vi "Write Node.vi"(8 "error in (no error)":errorcluster, 10 "BT.lvlib:abs_Node.lvclass":refnum<class "abs_Node.lvclass">, 11 "abs_Decorator in":refnum<class "abs_Decorator.lvclass">) -> (0 "error out":errorcluster, 3 "abs_Decorator out":refnum<class "abs_Decorator.lvclass">)   [LabVIEW 2021, in "BT.lvlib" / "abs_Decorator.lvclass"]
uses:
  abs_Decorator.lvclass
  abs_Node/abs_Node.lvclass
  abs_Decorator.lvclass/abs_Decorator.ctl
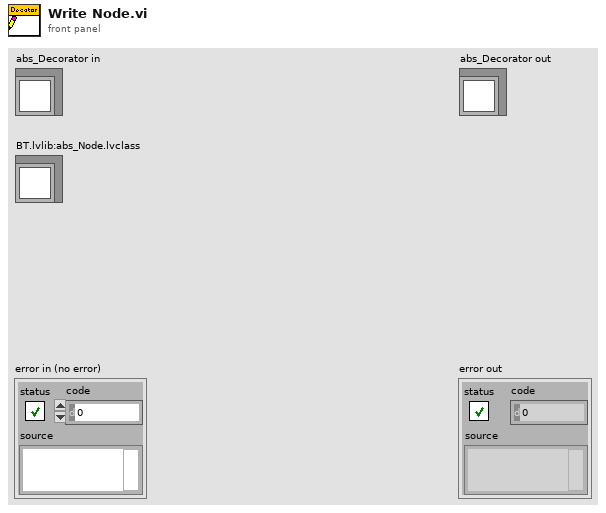
[diagram p1: front panel]
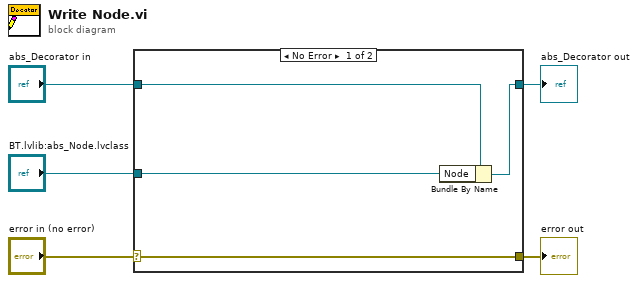
[diagram p0: block diagram]
diagram:
  n1 = case shown="No Error" "error in (no error)" {
    selector: "error in (no error)" -> [w9 w10]
    tunnel: [w9 w10] -> w4
    tunnel: [w7 w11] -> w2
    tunnel: "abs_Decorator in" -> [w8 w11]
    tunnel: "BT.lvlib:abs_Node.lvclass" -> [w6 _]
    frame No Error {
      n2 = Bundle By Name(cluster=w8, "Node"=w6) -> (w7:refnum<class "abs_Decorator.lvclass">)
    }
    frame Error {
    }
  }
  "error out" <- w4
  "abs_Decorator out" <- w2
